vi "Configure Advanced Trigger [AT] Core.vi"(7 "Trigger Slope (Positive)":i32(ring) caption="trigger slope (Positive)" items=["Positive", "Negative", "Either"], 8 "error in (no error)":errorcluster, 9 "Trigger Source (None)":string(combo) caption="trigger source (None)", 10 "Channel Name (\"\")":string="CHANNEL1" caption="channel name (\"CHANNEL1\")", 11 "CS++Fgen in":refnum<class "CS++Fgen.lvclass">) -> (0 "error out":errorcluster, 3 "CS++Fgen out":refnum<class "CS++Fgen.lvclass">)   [LabVIEW 2016, in "CS++Fgen.lvlib" / "CS++Fgen.lvclass"]
doc: "This VI configures the properties that control the function generator's advance trigger. These properties are the advance trigger source and slope.\n\nAn advance trigger advances generation to the end of the current waveform, where generation proceeds according to the current configuration.\n\nNote:\n\n(1) This VI is part of the IviFgenAdvanceTrigger [AT] extension group."
uses:
  CS++Fgen.lvclass
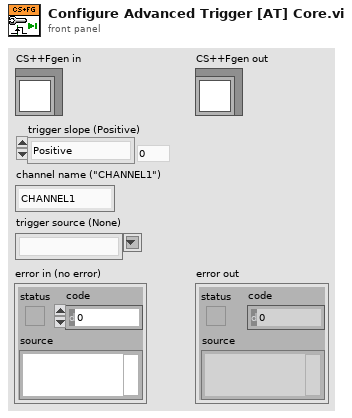
[diagram p1: front panel]
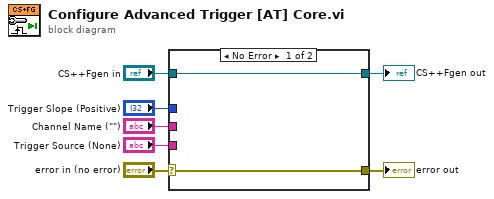
[diagram p0: block diagram]
diagram:
  n1 = case shown="No Error" "error in (no error)" {
    selector: "error in (no error)" -> [w8 w11]
    tunnel: [w8 w11] -> w6
    tunnel: [w9 w10] -> w4
    tunnel: "CS++Fgen in" -> [w9 w10]
    tunnel: "Trigger Slope (Positive)" -> [_ _]
    tunnel: "Channel Name (\"\")" -> [_ _]
    tunnel: "Trigger Source (None)" -> [_ _]
    frame No Error {
    }
    frame Error {
    }
  }
  "error out" <- w6
  "CS++Fgen out" <- w4
